vi "scaninput.vi"(8 "error in (no error)":errorcluster, 11 "6480 in":refnum<class "6480.lvclass">) -> (0 "error out":errorcluster, 3 "6480 out":refnum<class "6480.lvclass">)   [LabVIEW 2019, in "6480.lvclass"]
uses:
  6480.lvclass
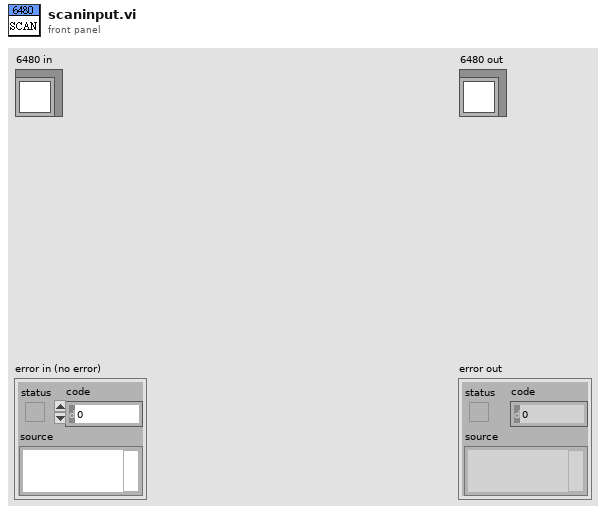
[diagram p1: front panel]
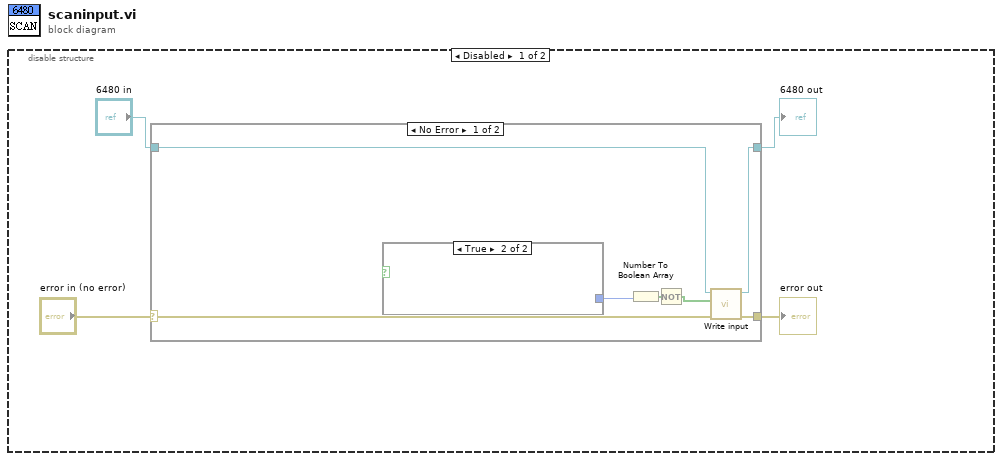
[diagram p0: block diagram]
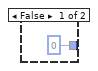
[diagram p2: hidden frame]
diagram:
  n1 = disable-structure shown="Disabled" {
    frame Disabled {
      n2 = case shown="No Error" "error in (no error)" {
        selector: "error in (no error)" -> [w7 w13]
        tunnel: "6480 in" -> [w11 w14]
        tunnel: [w10 w14] -> w2
        tunnel: [w6 w13] -> w1
        frame No Error {
          n3 = case shown="True" {
            selector: _ -> [_ _]
            tunnel: [u32 0 ("pIoState") _] -> w9
            frame False {
            }
            frame True {
            }
          }
          n4 = Number To Boolean Array(number=w9) -> (Boolean array=w8:bool[])
          n5 = Not(x=w8) -> (.not. x?=w5:bool[])
          n6 = call-dynamic "Write input.vi"("error in (no error)"=w7, "input"=w5, "IOCard in"=w11) -> ("error out"=w6:errorcluster, "IOCard out"=w10:refnum<class "6480.lvclass">)  [unwired: 7 in]
        }
        frame Error {
        }
      }
      "error out" <- w1
      "6480 out" <- w2
    }
    frame Enabled {
    }
  }
